vi "FolderDir.vi"(8 "error in (no error)":errorcluster, 11 "ImagePath":path=path "D:/Life/20191001_Accordance/Project/EPISIL/20200806-Camera/20200716/getimg_003.bmp") -> (0 "error out":errorcluster, 2 "ArrayTxt":string[](array[string]), 3 "ArrayImage":string[](array[string]))   [LabVIEW 2018]
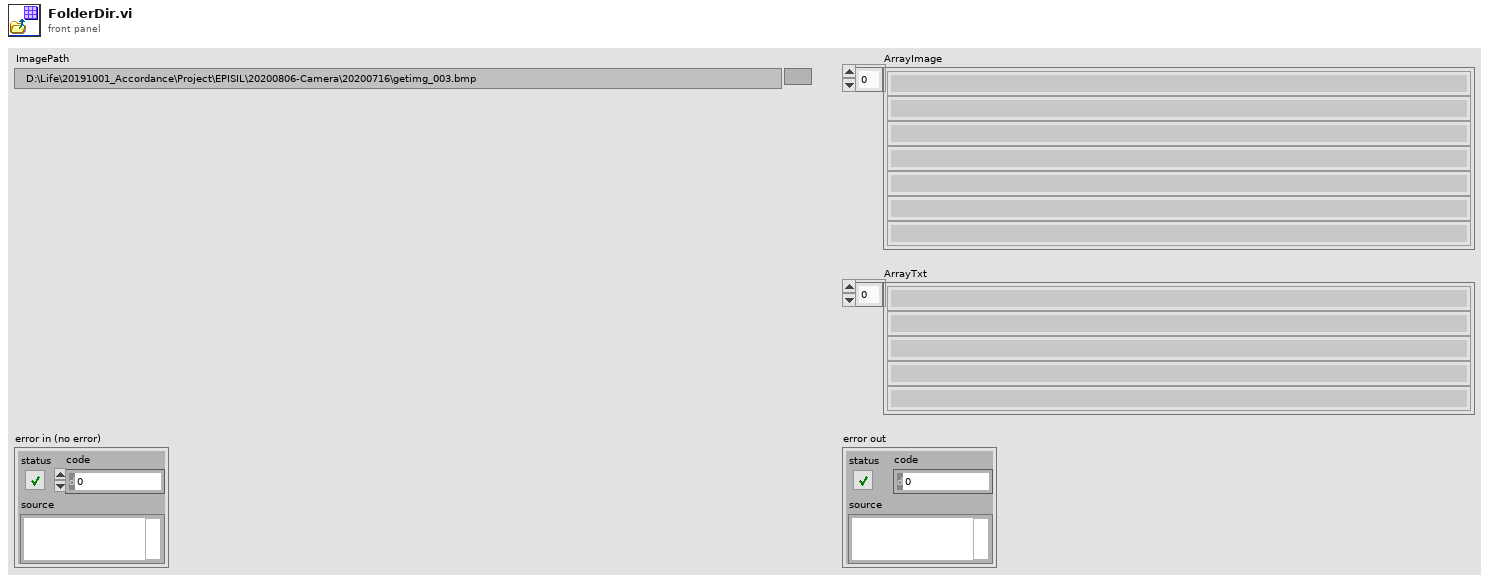
[diagram p1: front panel]
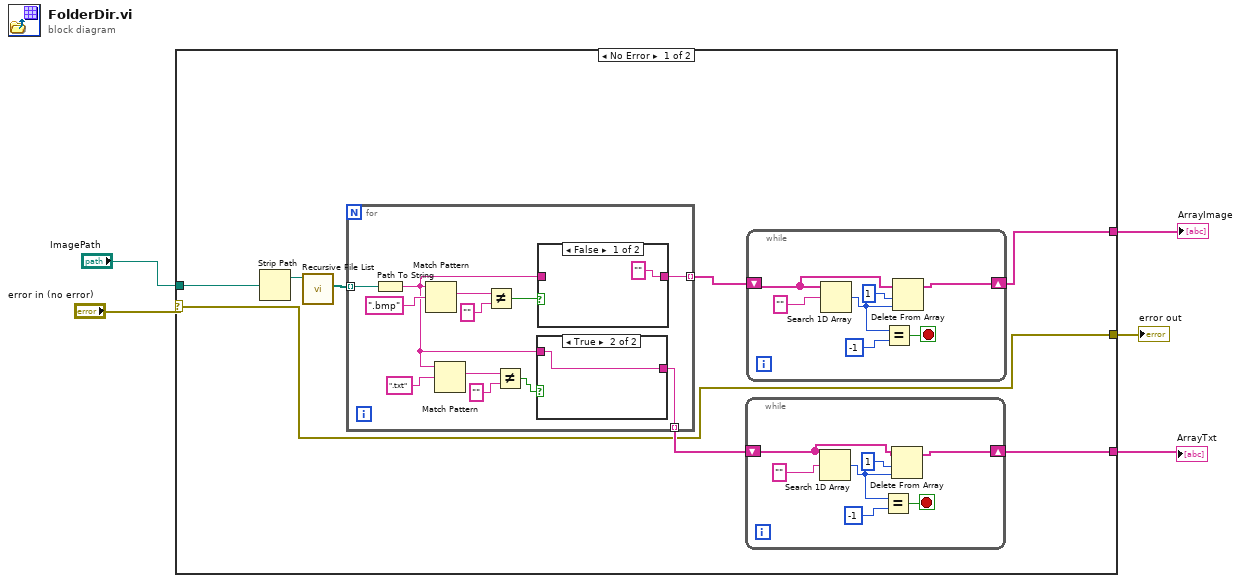
[diagram p0: block diagram]
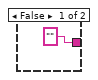
[diagram p2: hidden frame]
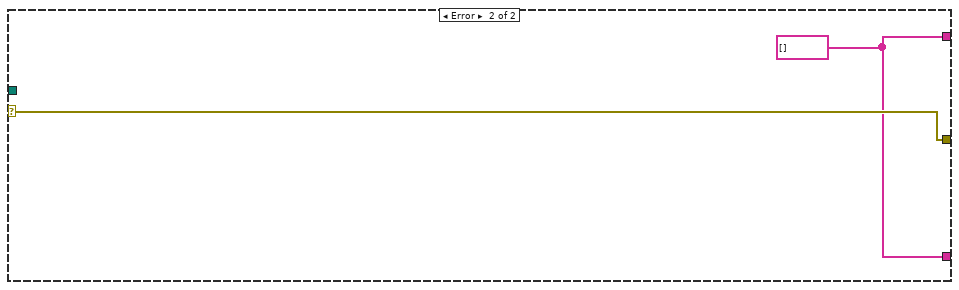
[diagram p4: hidden frame]
diagram:
  n1 = case shown="No Error" "error in (no error)" {
    selector: "error in (no error)" -> [w8 w45]
    tunnel: "ImagePath" -> [w9 _]
    tunnel: [w8 w45] -> w3
    tunnel: [w7 w44] -> w4
    tunnel: [w6 w44] -> w5
    frame No Error {
      n2 = Strip Path(path=w9) -> (stripped path=w12:path)  [unwired: 1 out]
      n3 = call <vilib>:"Recursive File List.vi"("Folder Path"=w12) -> ("All Files in Dir"=w13:path[])  [unwired: 6 in, 4 out]
      n4 = for {
        tunnel: w13 -> [w39] mode=indexing
        tunnel: [w34] -> w11 mode=indexing
        tunnel: [w28] -> w10 mode=indexing
        n5 = Path To String(path=w39) -> (string=w29:string)
        n6 = Match Pattern(string=w29, regular expression=".bmp") -> (match substring=w35:string)  [unwired: 1 in, 3 out]
        n7 = Match Pattern(string=w29, regular expression=".txt") -> (match substring=w31:string)  [unwired: 1 in, 3 out]
        n8 = Not Equal?(x=w35, y="") -> (x != y?=w37:bool)
        n9 = Not Equal?(x=w31, y="") -> (x != y?=w30:bool)
        n10 = case shown="True" w30 {
          tunnel: ["" w41] -> w28
          tunnel: w29 -> [_ w41]
          frame False {
          }
          frame True {
          }
        }
        n11 = case shown="False" w37 {
          tunnel: w29 -> [_ w43]
          tunnel: ["" w43] -> w34
          frame False {
          }
          frame True {
          }
        }
      }
      n12 = while {
        shift-right: [w19] -> w6
        shift-left: w10 -> [w15]
        stop <- w18 stop-if-true
        n13 = Search 1D Array(1D array=w15, element="") -> (index of element=w17:i32)  [unwired: 1 in]
        n14 = Equal?(x=w17, y=-1) -> (x = y?=w18:bool)
        n15 = Delete From Array(array=w15, length=1, index=w17) -> (array with subset deleted=w19:string[])  [unwired: 1 out]
      }
      n16 = while {
        shift-right: [w24] -> w7
        shift-left: w11 -> [w26]
        stop <- w23 stop-if-true
        n17 = Search 1D Array(1D array=w26, element="") -> (index of element=w22:i32)  [unwired: 1 in]
        n18 = Equal?(x=w22, y=-1) -> (x = y?=w23:bool)
        n19 = Delete From Array(array=w26, length=1, index=w22) -> (array with subset deleted=w24:string[])  [unwired: 1 out]
      }
    }
    frame Error {
      w44 = string[] []
    }
  }
  "error out" <- w3
  "ArrayImage" <- w4
  "ArrayTxt" <- w5
